vi "Memory.Pointer.Dispose.vi"(8 "error in (no error)":errorcluster, 11 "pointer":refnum<class "Memory.Pointer.lvclass">) -> (0 "error out":errorcluster, 3 "return":i32)   [LabVIEW 2016, in "Memory Manager.lvlib" / "Memory.Pointer.lvclass"]
uses:
  Memory.Pointer.lvclass
  Memory.Pointer.lvclass/Memory.Pointer.ctl
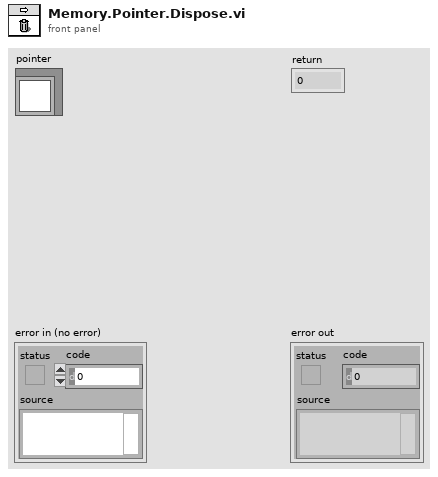
[diagram p1: front panel]
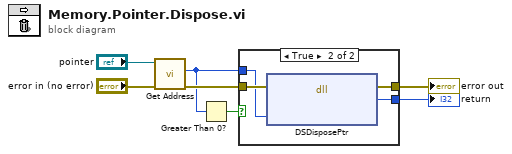
[diagram p0: block diagram]
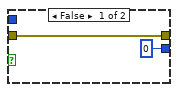
[diagram p2: hidden frame]
diagram:
  n1 = call "Get Address.vi"("error in (no error)"="error in (no error)", "Pointer in"="pointer") -> ("error out"=w7:errorcluster, "address"=w6:u64)  [unwired: 7 in, 1 out]
  n2 = Greater Than 0?(x=w6) -> (x > 0?=w5:bool)
  n3 = case shown="True" w5 {
    tunnel: w7 -> [w9 w13]
    tunnel: [w9 w12] -> w1
    tunnel: w6 -> [_ w11]
    tunnel: [0 ("return") w10] -> w2
    frame False {
    }
    frame True {
      n4 = dll-call lib="LabVIEW" fn="DSDisposePtr"(error in=w13, "pointer"=w11) -> (error out=w12:errorcluster, "return"=w10:i32)  [unwired: 3 in, 1 out]
    }
  }
  "error out" <- w1
  "return" <- w2
